vi "AccumulateData.vi"(6 "new block":T3, 7 "data group":string, 8 "error in (no error)":errorcluster, 9 "data in":T1, 11 "accumulation settings":T5) -> (0 "error out":errorcluster, 1 "pulse positions array":T2[](array[typedef]), 2 "waveforms":waveform(sgl)[](array[waveform]), 3 "accumulation settings out":T5, 4 "most recent map":T4, 5 "accumulation complete":bool)   [LabVIEW 2017, in "DataAccumulator.lvlib"]
uses:
  <vilib>/addons/InsightCM/Devices/Shared/Common/DataAccumulator/DataAccumulator.lvlib
  <vilib>/addons/InsightCM/Devices/Shared/Common/DVRBuffer/controls/BufferLocation.ctl
  <vilib>/addons/InsightCM/Devices/Shared/Common/DataAccumulator/controls/AccumulationSettings.ctl
  <vilib>/addons/InsightCM/Devices/Shared/Common/DataAccumulator/controls/accumulationType.ctl
  <vilib>/addons/InsightCM/Utilities/Analysis/Shared/controls/PulsePositions.ctl
  <vilib>/addons/PointValueMap/controls/PointMap.ctl
  <vilib>/addons/InsightCM/Devices/Shared/Common/DataAccumulator/controls/DataStoreType.ctl
  <vilib>/addons/InsightCM/Devices/Shared/Common/DVRBuffer/DVRBuffer.lvlib
  <vilib>/addons/PointValueMap/PointValueMap.lvlib
  <vilib>/addons/InsightCM/Utilities/Analysis/Shared/AnalysisHelper.lvlib
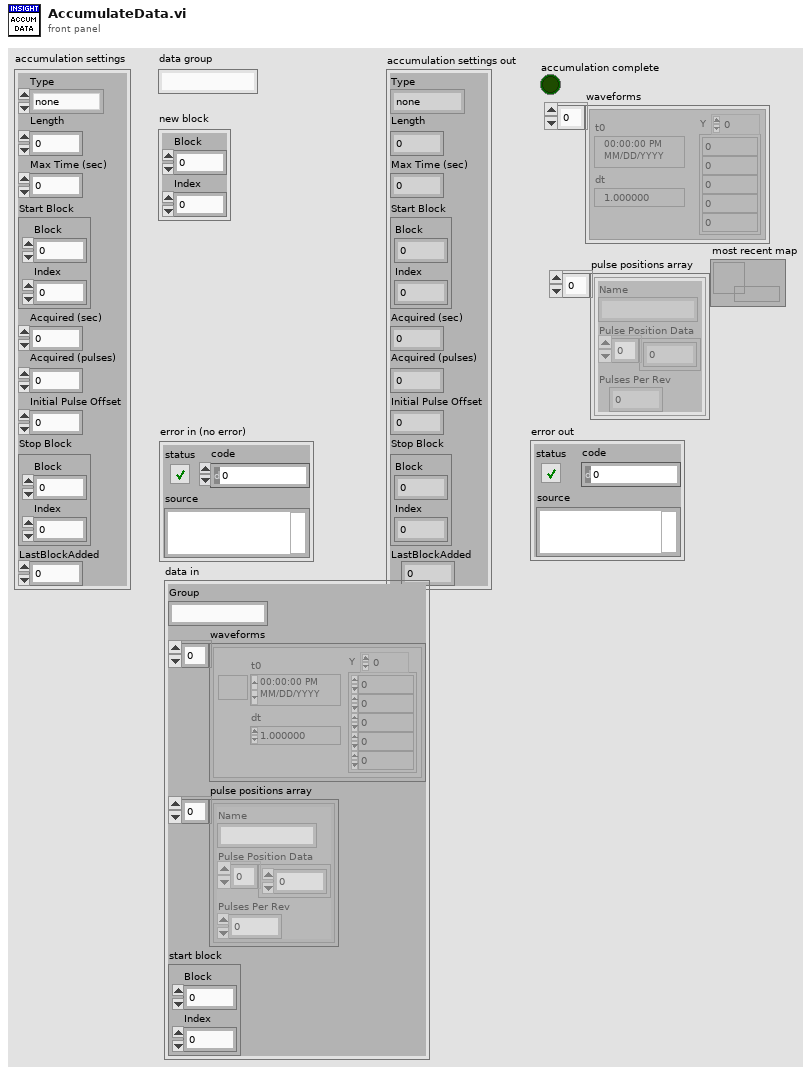
[diagram p1: front panel]
types:
  T1 = typedef "DataAccumulator.lvlib/DataStoreType.ctl" = cluster{"Group":string, "waveforms":waveform(sgl)[], "pulse positions array":T2[], "start block":T3}
  T2 = typedef "AnalysisHelper.lvlib/PulsePositions.ctl" = cluster{"Name":string, "Pulse Position Data":dbl[], "Pulses Per Rev":i32}
  T3 = typedef "DVRBuffer.lvlib/BufferLocation.ctl" = cluster{"Block":u32, "Index":i32}
  T4 = typedef "PointValueMap.lvlib/PointMap.ctl" = refnum<data-value>
  T5 = typedef "DataAccumulator.lvlib/AccumulationSettings.ctl" = cluster{"Type":T6, "Length":dbl, "Max Time (sec)":dbl, "Start Block":T3, "Acquired (sec)":dbl, "Acquired (pulses)":i32, "Initial Pulse Offset":dbl, "Stop Block":T3, "LastBlockAdded":u32}
  T6 = typedef "DataAccumulator.lvlib/accumulationType.ctl" = enum16{"none", "seconds", "revolutions"}
  T7 = typedef "DVRBuffer.lvlib/DVRElement.ctl" = cluster{"location":u32, "DVR":u32, "points":i32, "dt":dbl, "PulsePositions":dbl[], "Pulses Per Rev":dbl}
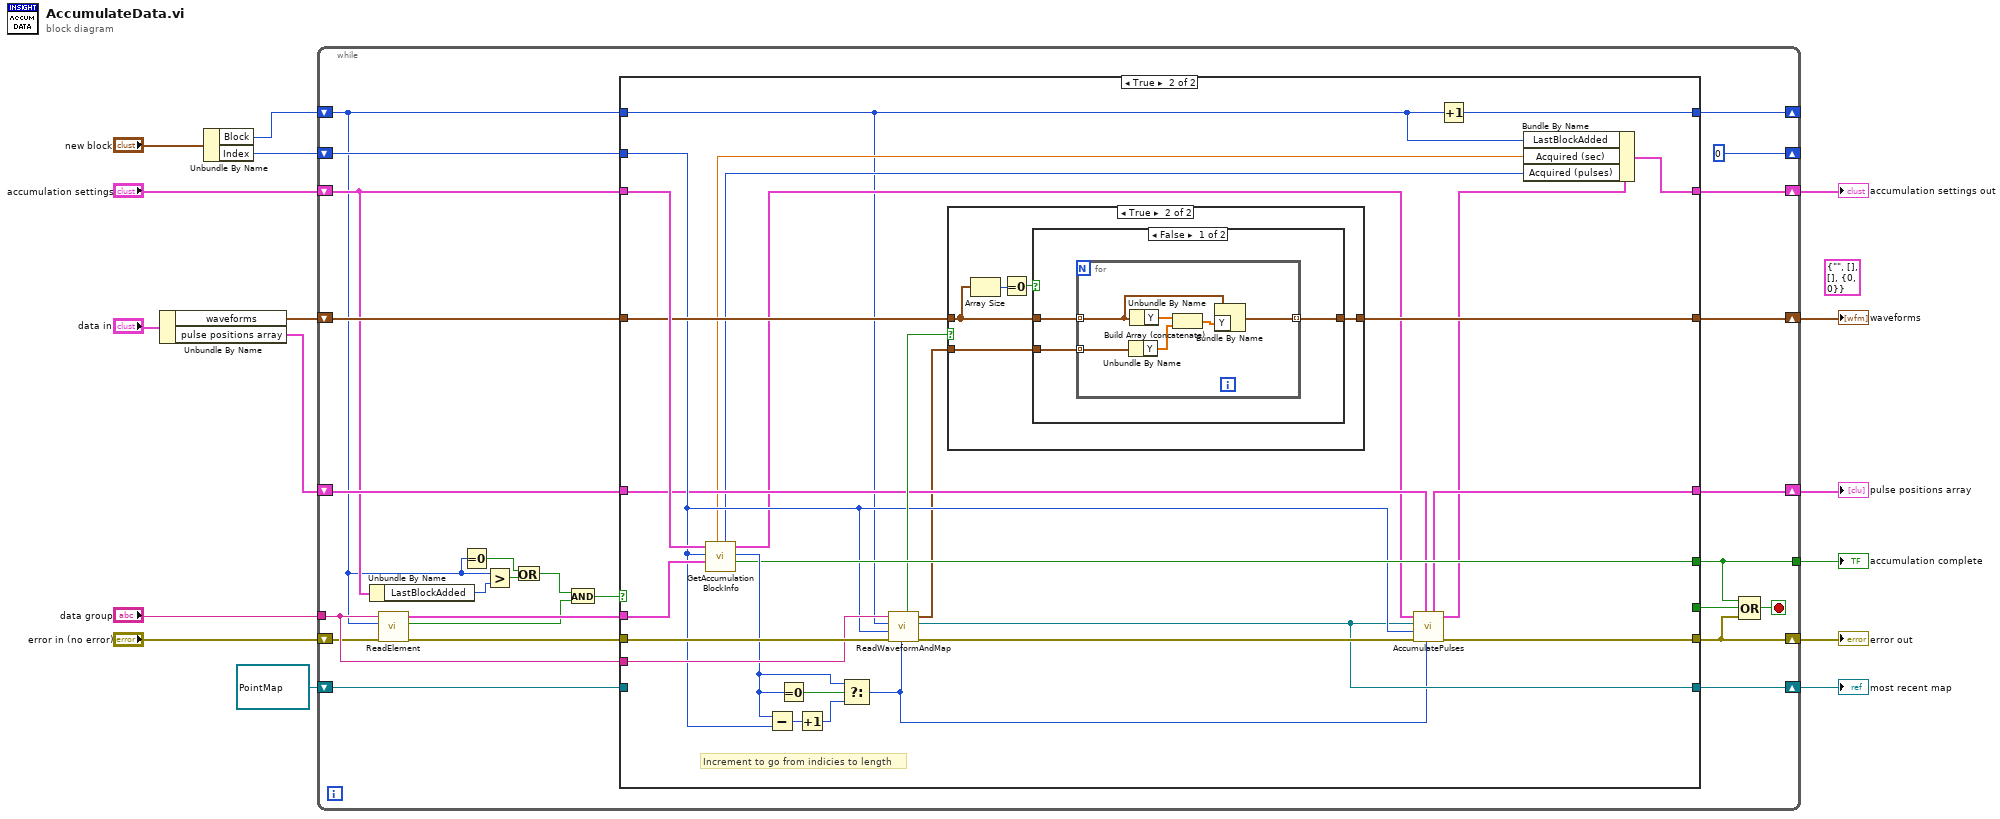
[diagram p0: block diagram]
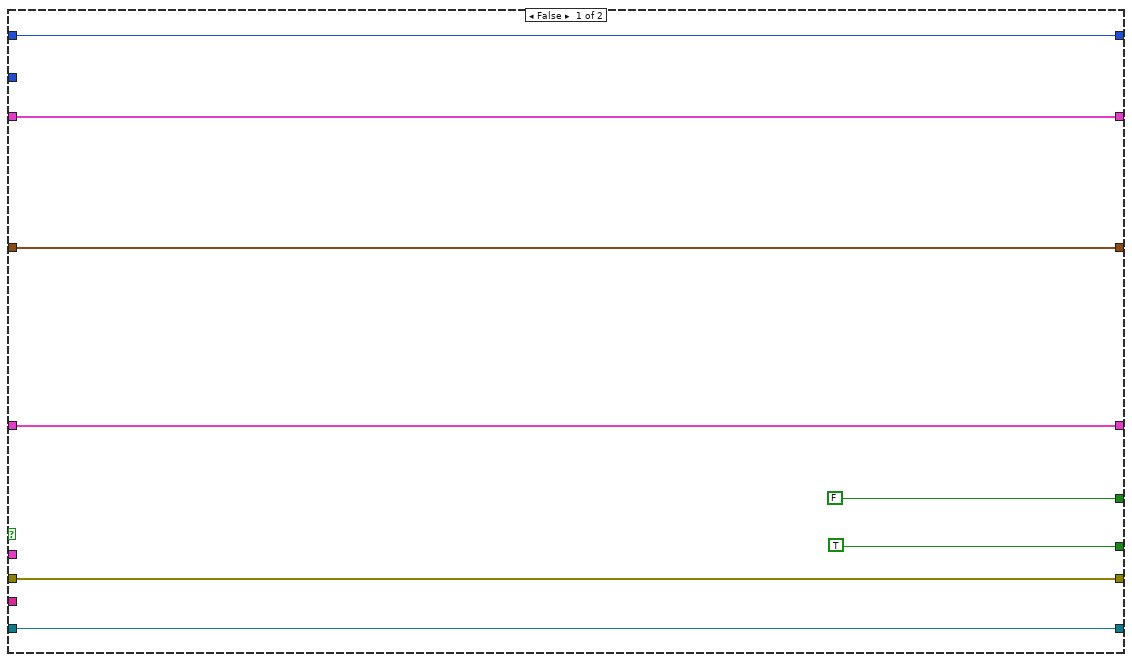
[diagram p2: hidden frame]
diagram:
  (unwired) T1 {"Group"="", "waveforms"=[], "pulse positions array"=[], "start block"={"Block"=0, "Index"=0}} ("data out")
  n1 = Unbundle By Name("data in") -> ("waveforms"=w2:waveform(sgl)[], "pulse positions array"=w1:T2[])
  n2 = Unbundle By Name("new block") -> ("Block"=w15:u32, "Index"=w14:i32)
  n3 = while {
    shift-right: [w39] -> _
    shift-left: w15 -> [w19]
    shift-right: [0 ("Index")] -> _
    shift-left: w14 -> [w37]
    tunnel: "data group" -> [w35]
    shift-right: [w36] -> w11
    shift-left: "accumulation settings" -> [w24]
    shift-right: [w33] -> w9
    shift-left: w2 -> [w34]
    tunnel: [w27] -> w10
    shift-right: [w31] -> w8
    shift-left: w1 -> [w32]
    shift-right: [w30] -> w6
    shift-left: "error in (no error)" -> [w29]
    shift-right: [w28] -> w5
    shift-left: T4 refnum ("map") -> [w25]
    stop <- w40 stop-if-true
    n4 = Unbundle By Name(w24) -> ("LastBlockAdded"=w21:u32)
    n5 = call <vilib>:"ReadElement.vi"("error in (no error)"=w29, "buffer location"=w19, "name"=w35) -> ("error out"=w42:errorcluster, "found"=w23:bool, "DVR element"=w41:T7)  [unwired: 6 in]
    n6 = Equal To 0?(x=w19) -> (x = 0?=w18:bool)
    n7 = Greater?(x=w19, y=w21) -> (0:w20:bool)
    n8 = Or(x=w18, y=w20) -> (x .or. y?=w17:bool)
    n9 = And(x=w17, y=w23) -> (x .and. y?=w22:bool)
    n10 = case shown="True" w22 {
      tunnel: w42 -> [w50 w74]
      tunnel: w41 -> [_ w75]
      tunnel: [w50 w64] -> w30
      tunnel: [w49 w53] -> w36
      tunnel: w24 -> [w49 w76]
      tunnel: [w48 w77] -> w39
      tunnel: w19 -> [w48 w51]
      tunnel: w37 -> [_ w63]
      tunnel: w35 -> [_ w73]
      tunnel: [FALSE ("condition met") w69] -> w27
      tunnel: w34 -> [w47 w67]
      tunnel: [w47 w66] -> w33
      tunnel: w32 -> [w45 w62]
      tunnel: [w45 w61] -> w31
      tunnel: [w43 w59] -> w28
      tunnel: [TRUE ("condition met") _] -> w26
      tunnel: w25 -> [w43 _]
      frame False {
      }
      frame True {
        # "Increment to go from indicies to length"
        n11 = call <vilib>:"GetAccumulationBlockInfo.vi"("block"=w75, "start index"=w63, "accumulation settings"=w76) -> ("condition met"=w69:bool, "stop index (include)"=w71:i32, "updated accumulation settings"=w60:T5, "acquired (pulses)"=w55:i32, "acquired (sec)"=w56:dbl)  [unwired: 4 in]
        n12 = Subtract(x=w71, y=w63) -> (x-y=w70:i32)
        n13 = Equal To 0?(x=w71) -> (x = 0?=w72:bool)
        n14 = Increment(x=w70) -> (x+1=w58:i32)
        n15 = Select(t=w71, s=w72, f=w58) -> (s? t:f=w57:i32)
        n16 = call <vilib>:"ReadWaveformAndMap.vi"("length"=w57, "error in (no error)"=w74, "index"=w63, "buffer location"=w51, "data group"=w73) -> ("error out"=w65:errorcluster, "map"=w59:T4, "waveforms"=w52:waveform(sgl)[], "found"=w68:bool)  [unwired: 2 in, 1 out]
        n17 = case shown="True" w68 {
          tunnel: w52 -> [_ w80]
          tunnel: w67 -> [w78 w79]
          tunnel: [w78 w81] -> w66
          frame False {
          }
          frame True {
            n18 = Array Size(array=w79) -> (size(s)=w83:i32)
            n19 = Equal To 0?(x=w83) -> (x = 0?=w82:bool)
            n20 = case shown="False" w82 {
              tunnel: [w84 w93] -> w81
              tunnel: w80 -> [w85 w93]
              tunnel: w79 -> [w86 _]
              frame False {
                n21 = for {
                  tunnel: w86 -> [w88] mode=indexing
                  tunnel: w85 -> [w92] mode=indexing
                  tunnel: [w87] -> w84 mode=indexing
                  n22 = Unbundle By Name(w92) -> ("Y"=w90:sgl[])
                  n23 = Unbundle By Name(w88) -> ("Y"=w91:sgl[])
                  n24 = Build Array (concatenate)(w91, w90) -> (w89:sgl[])
                  n25 = Bundle By Name(cluster=w88, "Y"=w89) -> (w87:waveform(sgl))
                }
              }
              frame True {
              }
            }
          }
        }
        n26 = call <vilib>:"AccumulatePulses.vi"("length"=w57, "pulse positions array"=w62, "error in (no error)"=w65, "index"=w63, "map"=w59, "accumulation settings"=w60) -> ("error out"=w64:errorcluster, "accumulation settings"=w54:T5, "pulse positions array"=w61:T2[])  [unwired: 3 in]
        n27 = Increment(x=w51) -> (x+1=w77:u32)
        n28 = Bundle By Name(cluster=w54, "LastBlockAdded"=w51, "Acquired (sec)"=w56, "Acquired (pulses)"=w55) -> (w53:T5)
      }
    }
    n29 = Compound Arithmetic op=OR(w27, w26, w30) -> (w40:bool)
  }
  "accumulation settings out" <- w11
  "accumulation complete" <- w10
  "waveforms" <- w9
  "pulse positions array" <- w8
  "error out" <- w6
  "most recent map" <- w5
